vi "Subvi sample and hold U16.vi"(8 "Clock":bool, 9 "Input":u16) -> (1 "Output":u16)   [LabVIEW 2017]
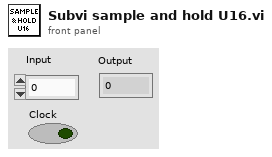
[diagram p1: front panel]
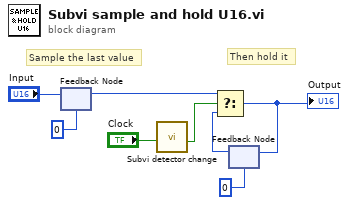
[diagram p0: block diagram]
diagram:
  # "Then hold it"
  # "Sample the last value"
  n1 = feedback #1(u16 0) -> (w5:u16)
  n2 = feedback-in #1("Input") -> ()
  n3 = call "Subvi detector change.vi"("Input"="Clock") -> ("Output"=w1:bool)  [unwired: 8 in]
  n4 = feedback #2(u16 0) -> (w4:u16)
  n5 = Select(t=w5, s=w1, f=w4) -> (s? t:f=w3:u16)
  "Output" <- w3
  n6 = feedback-in #2(w3) -> ()
